vi "RSZVB Set TDIF Compensation State.vi"(8 "error in (no error)":errorcluster {"code" format="%.0x"}, 9 "Compensation State (F: Off)":bool, 10 "Channel (1)":i32=1, 11 "VISA session":refnum<visa-resource-name>) -> (0 "error out":errorcluster {"code" format="%.0x"}, 3 "dup VISA session":refnum<visa-resource-name>)   [LabVIEW 2011]
doc: "This VI selects the calculation method for S-parameters, ratios and derived quantities during an amplitude imbalance or phase imbalance sweep.\n\nNote(s):\n\n(1) This VI is available only with option R&S ZVA-K6 and ZVT instrument.\n\nRemote-control command(s):\nCALCulate<Ch>:TDIF:IMBalance:COMPensation[:STATe] <Boolean>"
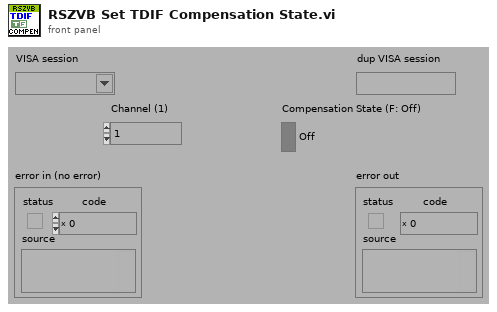
[diagram p1: front panel]
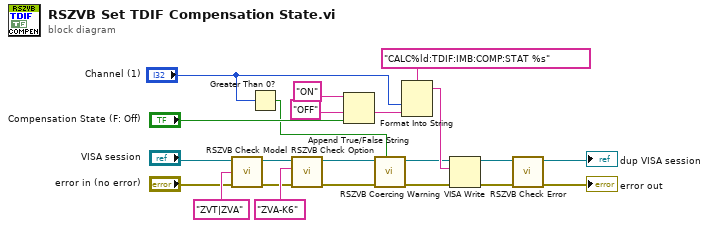
[diagram p0: block diagram]
diagram:
  n1 = call "RSZVB Check Model.vi"("error in (no error)"="error in (no error)", "Model"="ZVT|ZVA" ("Options"), "VISA session"="VISA session") -> ("error out"=w13:errorcluster, "dup VISA session"=w14:refnum<visa-resource-name>)  [unwired: 7 in]
  n2 = Greater Than 0?(x="Channel (1)") -> (x > 0?=w1:bool)
  n3 = call "RSZVB Check Option.vi"("error in (no error)"=w13, "Options"="ZVA-K6", "VISA session"=w14) -> ("error out"=w2:errorcluster, "dup VISA session"=w3:refnum<visa-resource-name>)  [unwired: 7 in]
  n4 = Append True/False String(1:"Compensation State (F: Off)", 2:"OFF", 3:"ON") -> (0:w7:string)  [unwired: 1 in]
  n5 = call "RSZVB Coercing Warning.vi"("In Range?"=w1, "error in (no error)"=w2, "VISA session"=w3) -> ("error out"=w5:errorcluster, "dup VISA session"=w4:refnum<visa-resource-name>)  [unwired: 7 in]
  n6 = Format Into String(format string="CALC%ld:TDIF:IMB:COMP:STAT %s", "Channel (1)", w7) -> (resulting string=w19:string)  [unwired: 2 in, 1 out]
  n7 = VISA Write(VISA resource name=w4, write buffer=w19, error in (no error)=w5) -> (VISA resource name out=w20:refnum<visa-resource-name>, error out=w21:errorcluster)  [unwired: 1 out]
  n8 = call "RSZVB Check Error.vi"("error in (no error)"=w21, "VISA session"=w20) -> ("error out"=→"error out":errorcluster, "dup VISA session"=→"dup VISA session":refnum<visa-resource-name>)  [unwired: 8 in]
